vi "rename IPF.vi"(8 "error in":errorcluster, 9 "APG Config":T1, 10 "Programs List":i32(listbox), 11 "ref.Program List":refnum<vi>) -> (0 "error out":errorcluster, 2 "new filename":string)   [LabVIEW 2013, in "Manipulate IPF.lvlib"]
uses:
  Manipulate IPF.lvlib
  Settings/type_def/APG Config.ctl
  Pack Data/type_def/file types.ctl
  <userlib>/_OpenG.lib/file/file.llb/Strip Path Extension - 1D Array of Strings__ogtk.vi
  3013/code/Modules/GUI/GUI_5/subPanels/program/program.lvlib
  <userlib>/_OpenG.lib/file/file.llb/Convert File Extension (String)__ogtk.vi
  3013/code/a3Di.lvlib
  <userlib>/_OpenG.lib/file/file.llb/Convert File Extension (Path)__ogtk.vi
  Pack Data/Pack Files.lvlib
  Pack Data/type_def/command.ctl
  Settings/APG_settings.lvlib
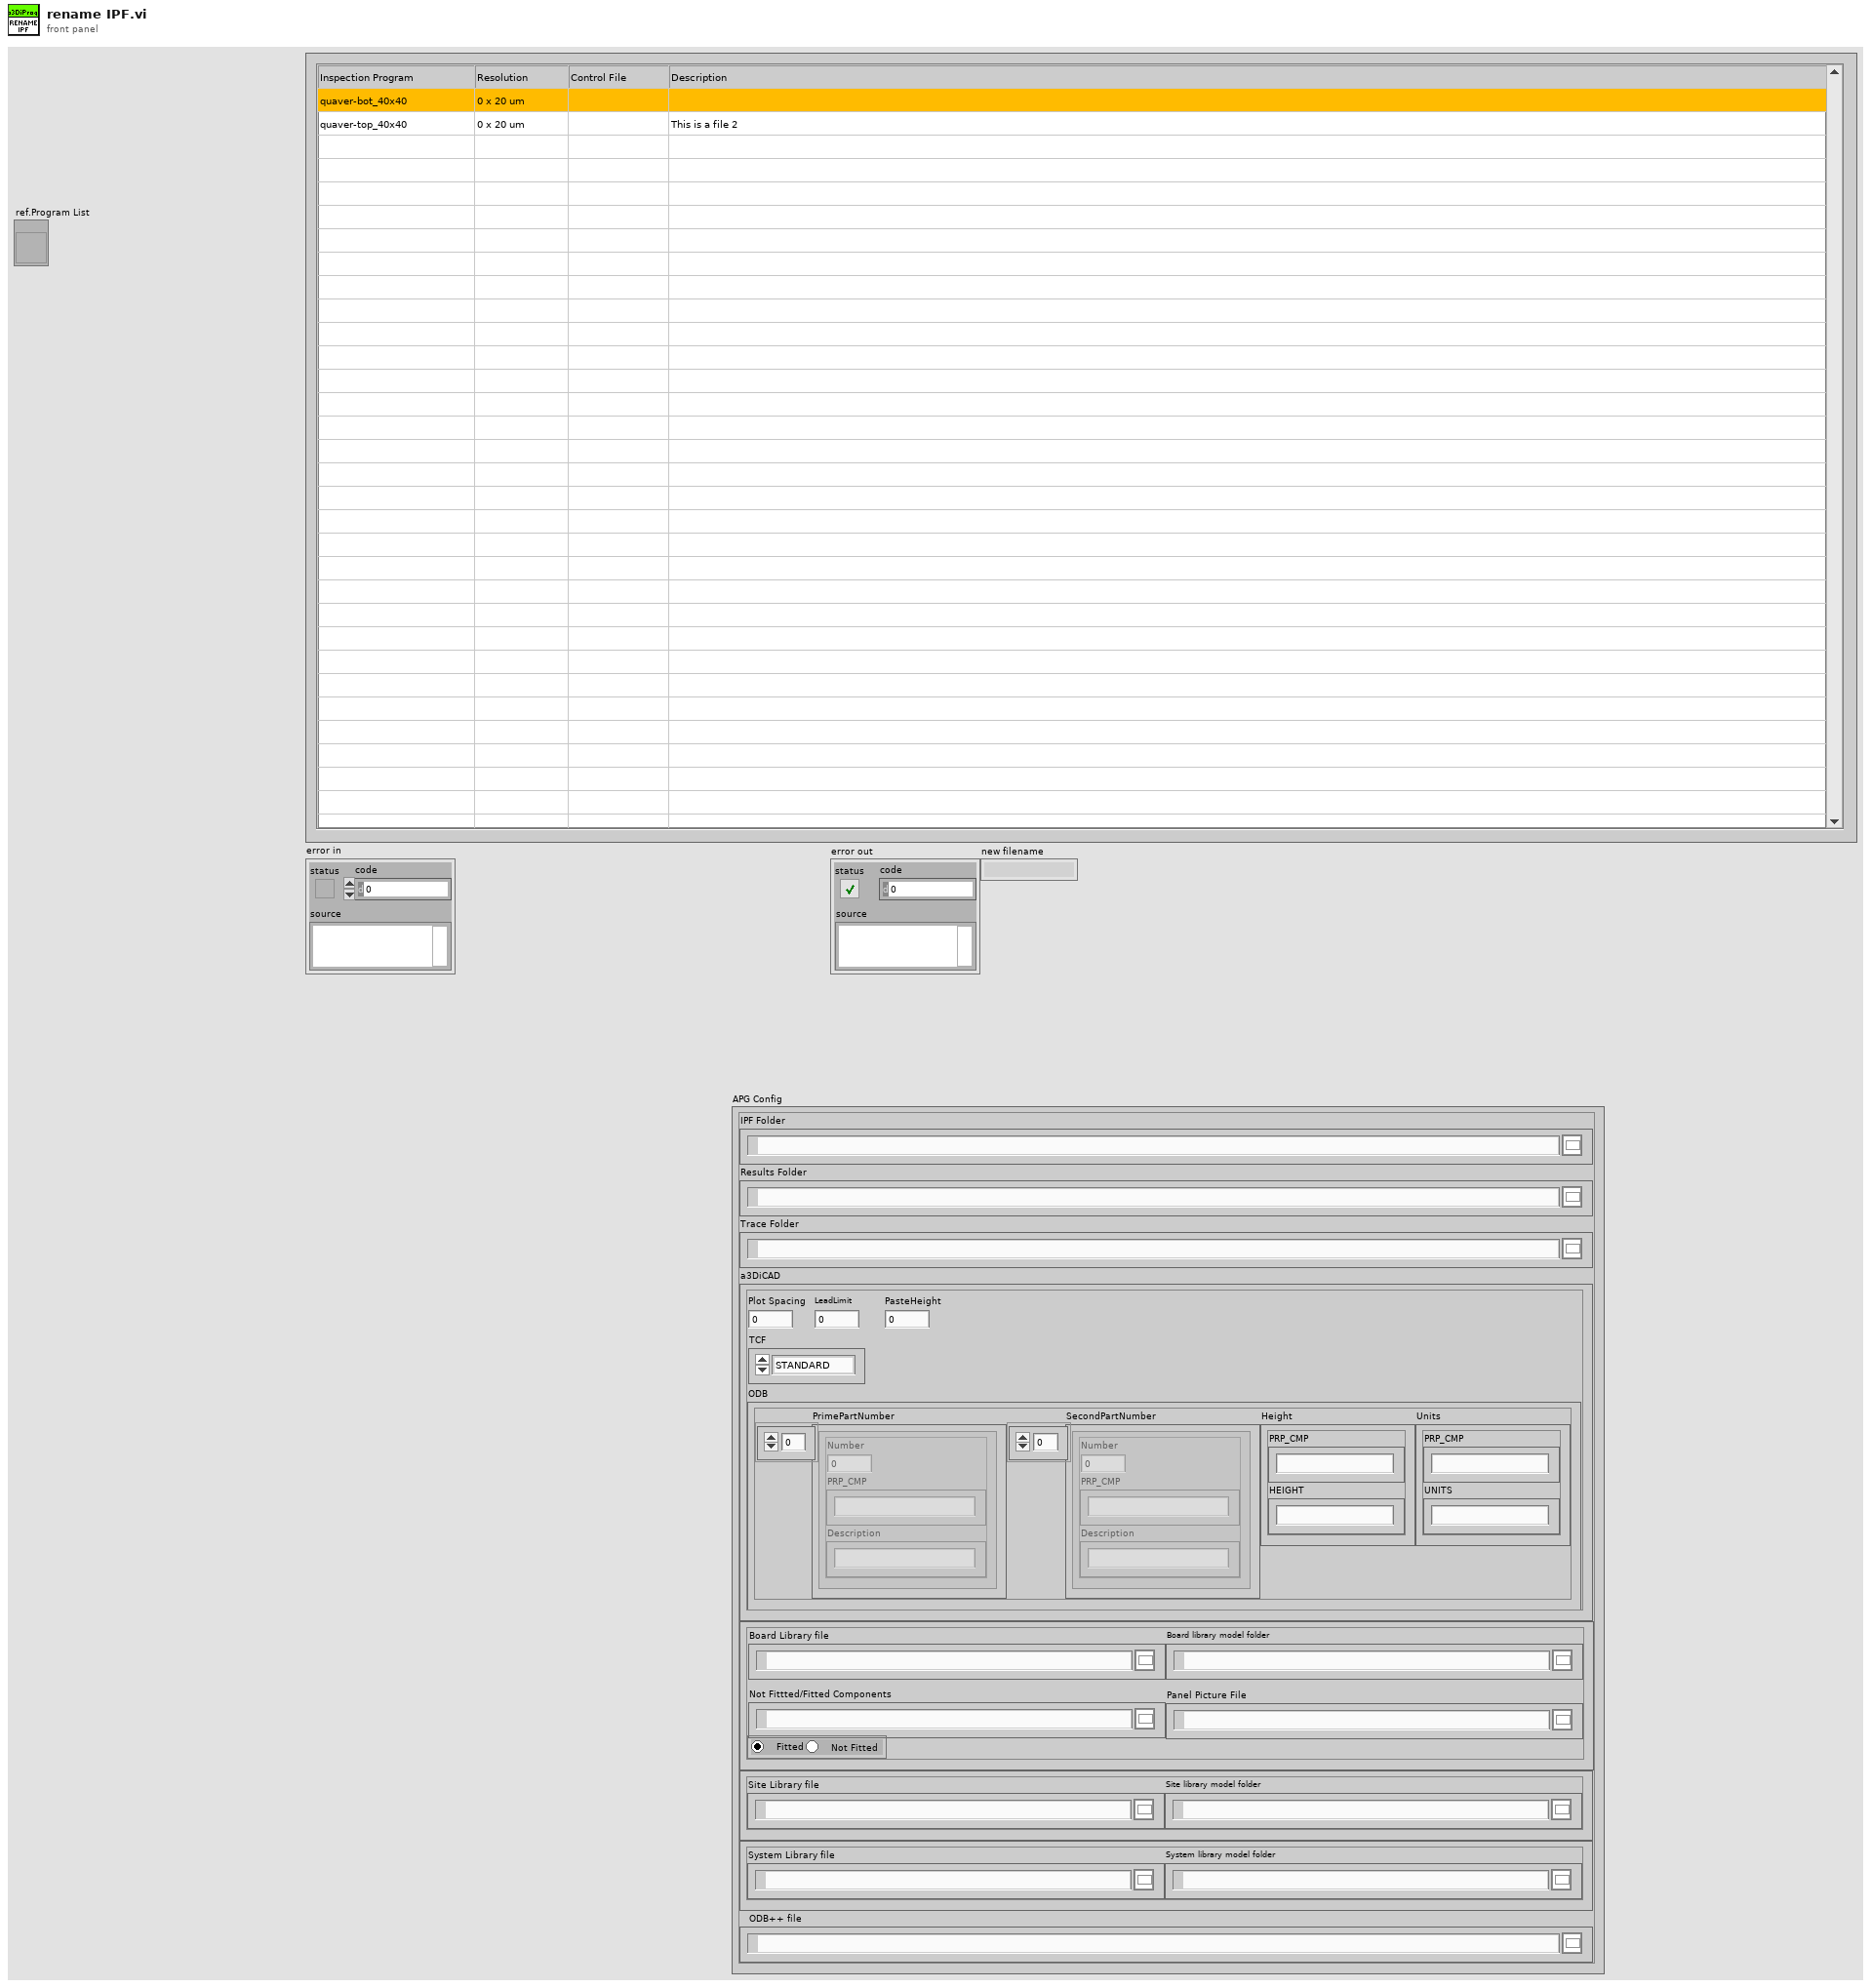
[diagram p1: front panel]
types:
  T1 = typedef "APG_settings.lvlib/APG Config.ctl" = cluster{"IPF Folder":path, "Results Folder":path, "Trace Folder":path, "a3DiCAD":cluster{"Plot Spacing":dbl, "TCF":enum16{"STANDARD", "PASTE", "LEAD"}, "LeadLimit":u32, "a3DiCADDebug":bool, "ODB":cluster{"PrimePartNumber":cluster{"Number":u32, "PRP_CMP":string, "Description":string}[], "SecondPartNumber":cluster{"Number":u32, "PRP_CMP":string, "Description":string}[], "Height":cluster{"PRP_CMP":string, "HEIGHT":string}, "Units":cluster{"PRP_CMP":string, "UNITS":string}}, "PasteHeight":dbl}, "a3DiCADcfg":path, "Board Library":cluster{"Board Library file":path, "Board library model folder":path, "Not Fittted/Fitted Components":path, "Panel Picture File":path, "Components":enum32{"Fitted", "Not Fitted "}}, "Site Library":cluster{"Site Library file":path, "Site library model folder":path}, "System Library":cluster{"System Library file":path, "System library model folder":path}, "ODB++ file":path}
  T2 = typedef "Pack Files.lvlib/file types.ctl" = enum16{"ODB", "TCF", "CAD Outline", "Config", "Inspection Prog", "a3Di-bin", "Results", "CAD Labels", "CAD Pads", "calScan_fid", "calScan_cal-tab", "PCB_SerialNumber", "CAD_Assembly", "Version", "Old Results", "CAD Picture", "Old TCF"}
  T3 = typedef "Pack Files.lvlib/command.ctl" = enum16{"Write", "Tar contents", "Read from Tar to File", "Delete", "Clean up Tar"}
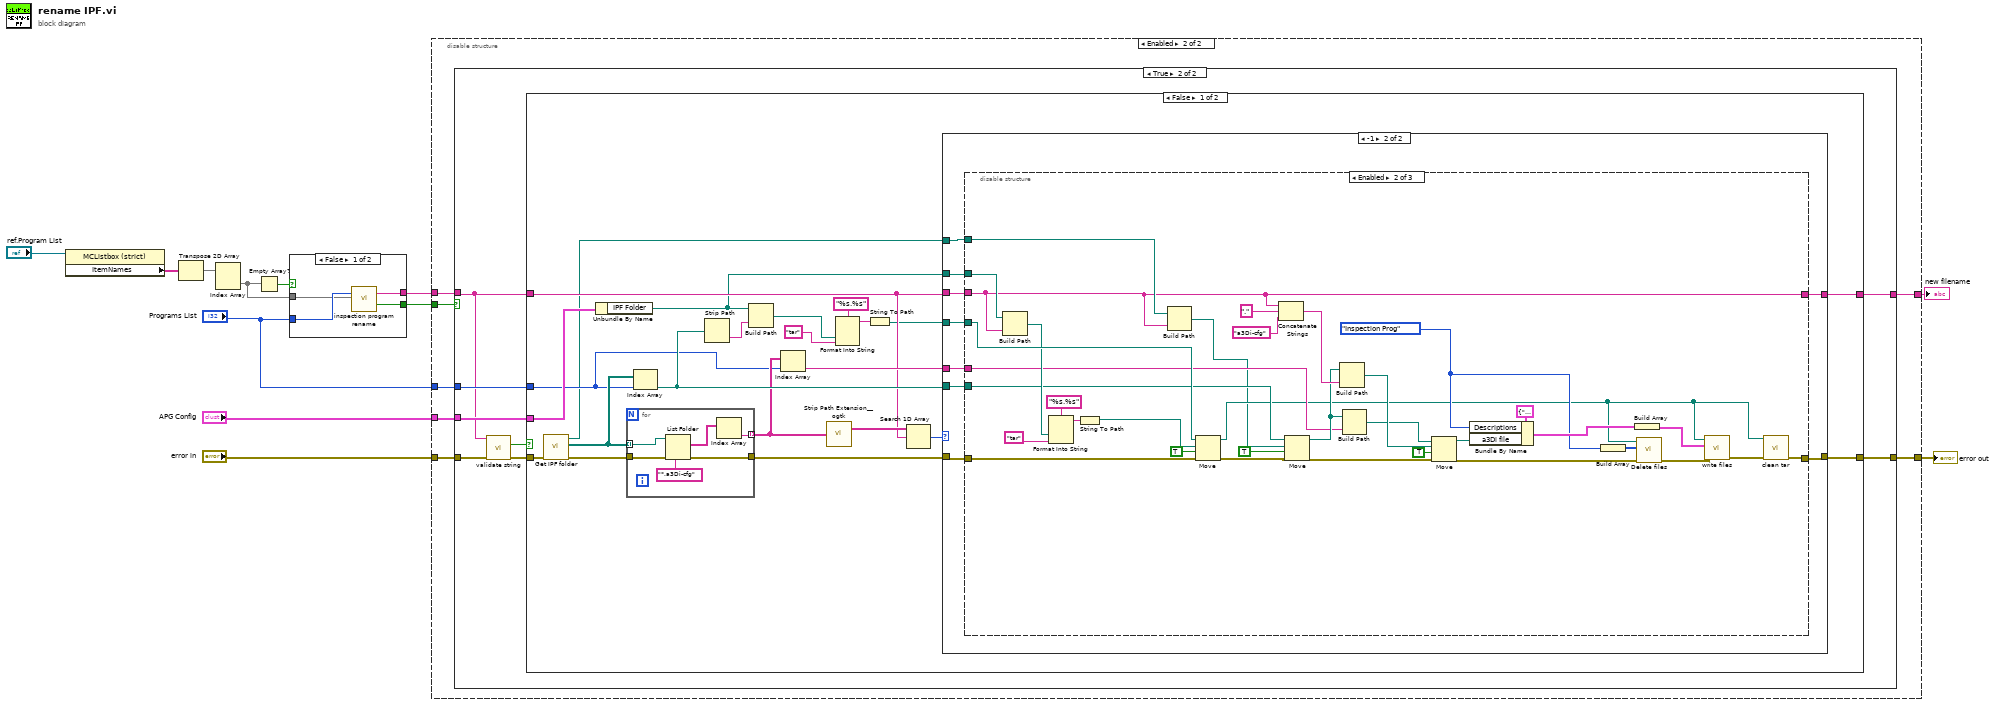
[diagram p0: block diagram]
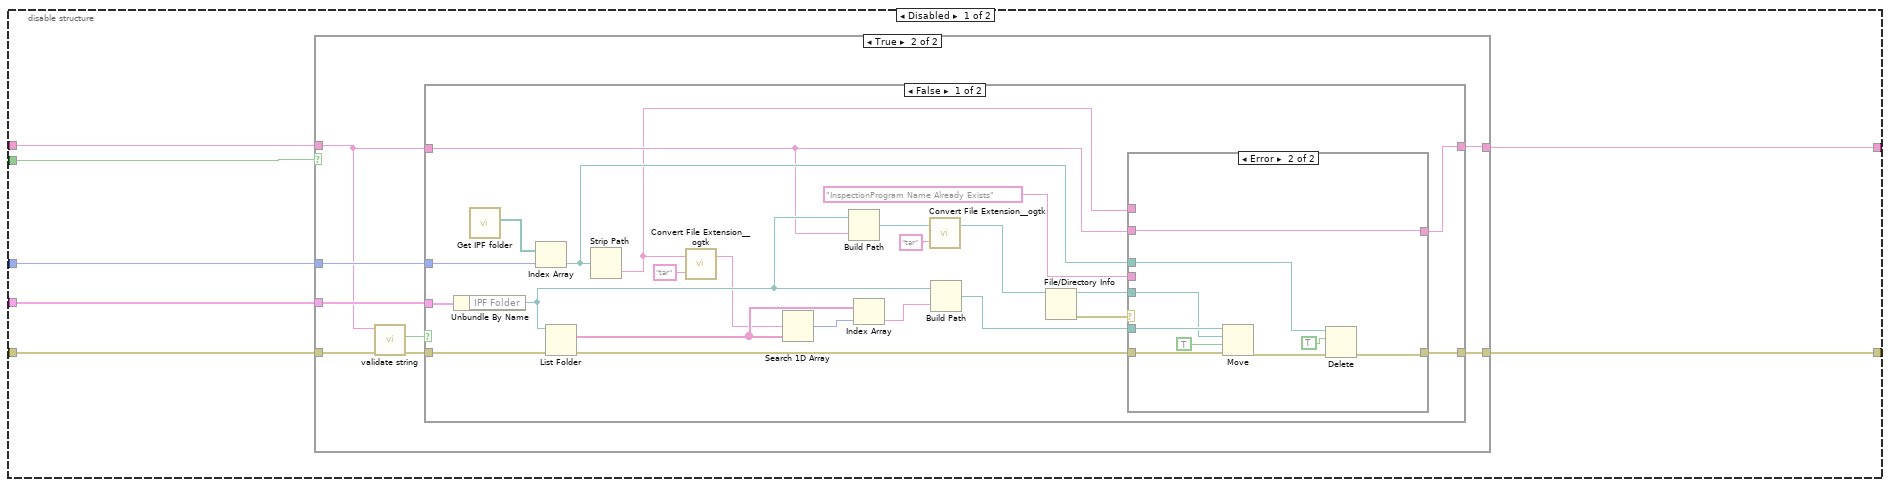
[diagram p2: hidden frame]
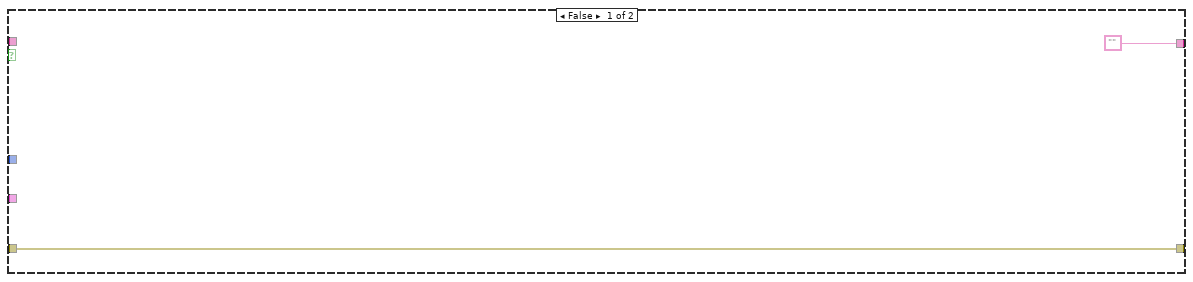
[diagram p3: hidden frame]
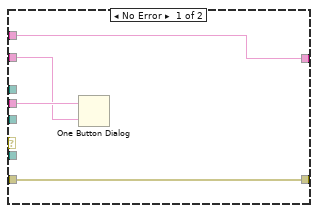
[diagram p4: hidden frame]
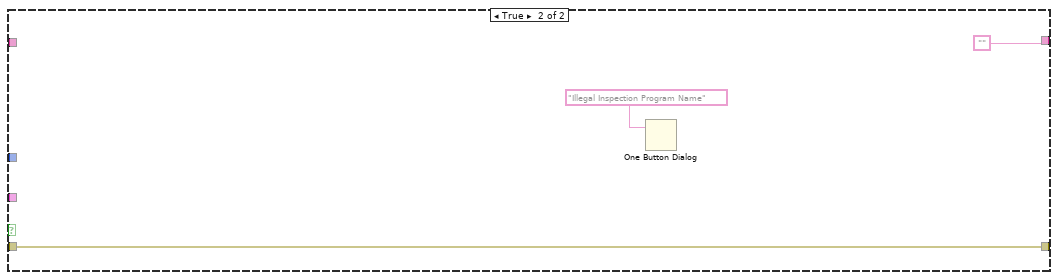
[diagram p5: hidden frame]
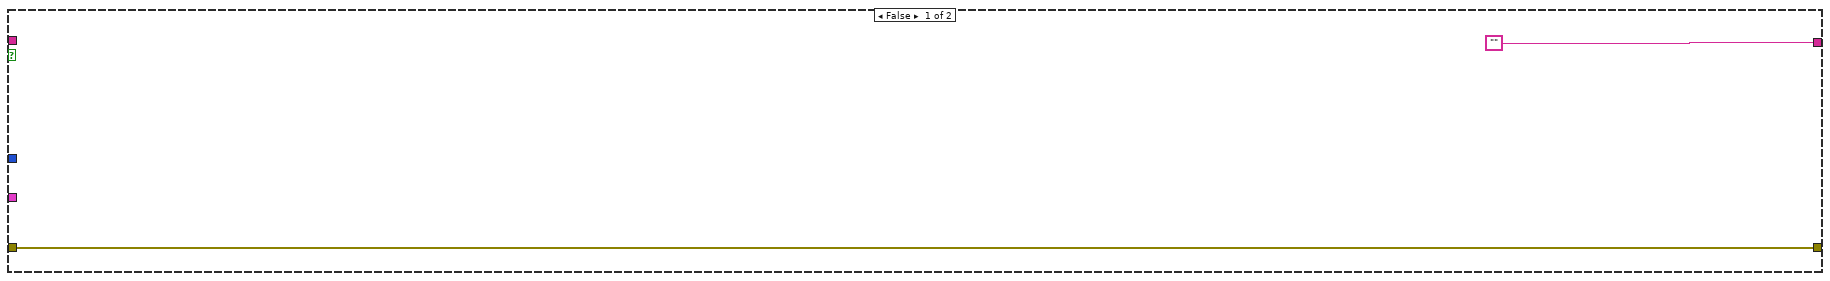
[diagram p6: hidden frame]
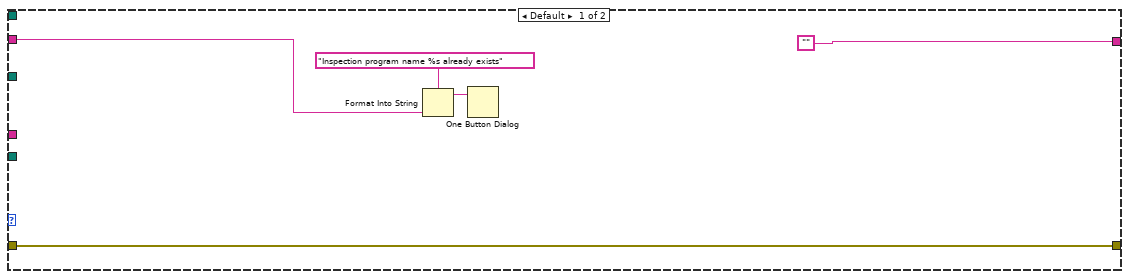
[diagram p7: hidden frame]
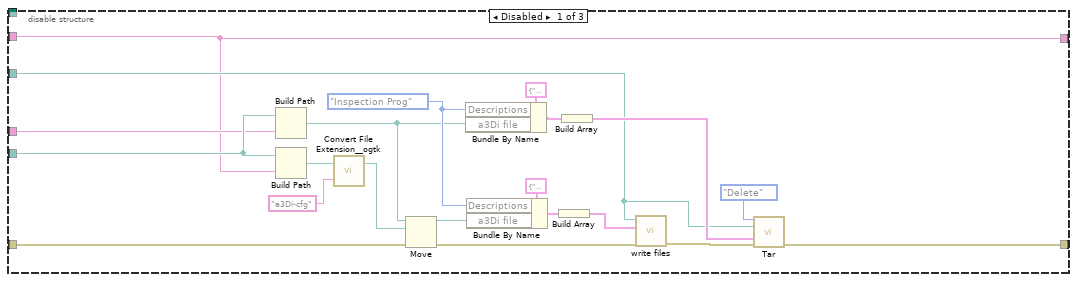
[diagram p8: hidden frame]
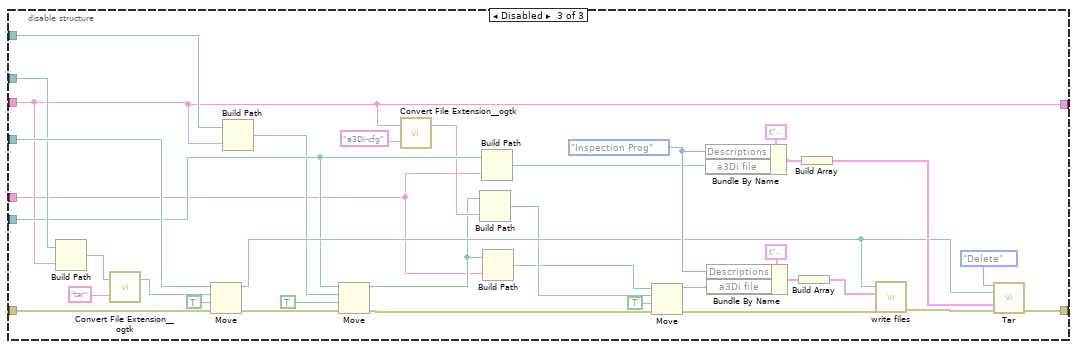
[diagram p9: hidden frame]
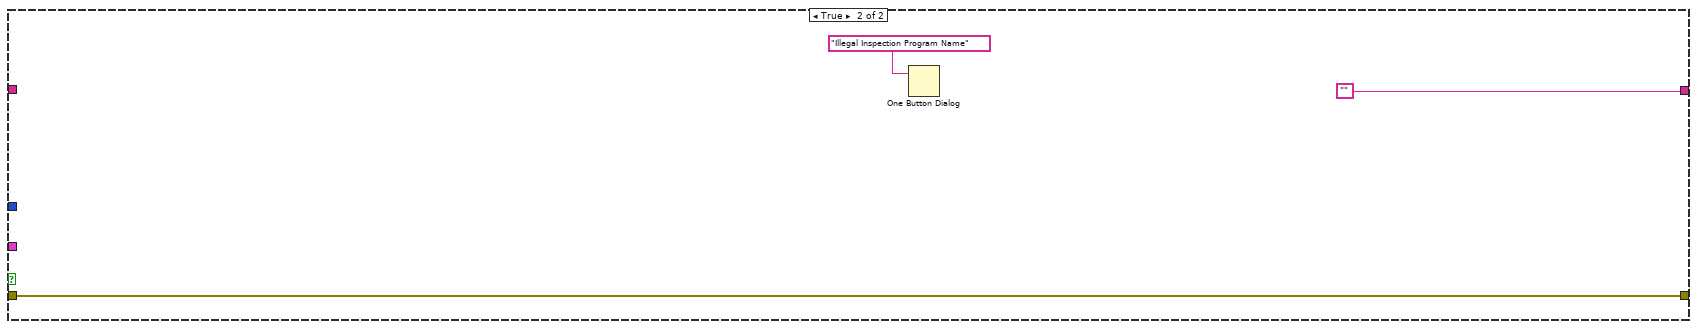
[diagram p10: hidden frame]
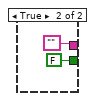
[diagram p11: hidden frame]
diagram:
  n1 = property class="MCListbox (strict)"(reference="ref.Program List") -> ("ItemNames"=w7:string[][])  [unwired: 1 in, 2 out]
  n2 = Transpose 2D Array(2D array=w7) -> (transposed array=w8:string[][])
  n3 = Index Array(array=w8) -> (element=w4:string[])  [unwired: 2 in]
  n4 = Empty Array?(array=w4) -> (empty?=w6:bool)
  n5 = case shown="False" w6 {
    tunnel: "Programs List" -> [w16 _]
    tunnel: w4 -> [w15 _]
    tunnel: [w14 FALSE ("OK")] -> w3
    tunnel: [w13 ""] -> w2
    frame False {
      n6 = call "inspection program rename.vi"("Selected Inspection Prog File Index"=w16, "Progs List[]"=w15) -> ("New Name"=w13:string, "OK"=w14:bool)  [unwired: 15 in, 1 out]
    }
    frame True {
    }
  }
  n7 = disable-structure shown="Enabled" {
    disable-tunnel: "error in" -> [w25 w81]
    disable-tunnel: [w24 w80] -> w11
    disable-tunnel: "APG Config" -> [w23 w79]
    disable-tunnel: "Programs List" -> [w22 w78]
    disable-tunnel: w3 -> [w21 w77]
    disable-tunnel: w2 -> [w20 w76]
    disable-tunnel: [w19 w75] -> w1
    frame Disabled {
      n8 = case shown="True" w21 {
        tunnel: w25 -> [w27 w33]
        tunnel: [w27 w35] -> w24
        tunnel: w23 -> [_ w32]
        tunnel: w22 -> [_ w34]
        tunnel: w20 -> [_ w29]
        tunnel: ["" w28] -> w19
        frame False {
        }
        frame True {
          n9 = call "validate string.vi"("error in (no error)"=w33, "String In"=w29) -> ("error out"=w30:errorcluster, "String Modified"=w31:bool)  [unwired: 6 in, 2 out]
          n10 = case shown="False" w31 {
            tunnel: [w58 w73] -> w35
            tunnel: w34 -> [w50 _]
            tunnel: w32 -> [w49 _]
            tunnel: w30 -> [w48 w73]
            tunnel: w29 -> [w38 _]
            tunnel: [w37 ""] -> w28
            frame False {
              n11 = Unbundle By Name(w49) -> ("IPF Folder"=w47:path)
              n12 = call "Get IPF folder.vi"() -> ("IPF sub folders"=w57:path[])  [unwired: 6 in, 5 out]
              n13 = Index Array(array=w57, index=w50) -> (element=w42:path)
              n14 = List Folder(path=w47, error in=w48) -> (filenames=w54:string[], error out=w55:errorcluster)  [unwired: 2 in, 2 out]
              n15 = Strip Path(path=w42) -> (name=w36:string)  [unwired: 1 out]
              n16 = call-poly <userlib>:"Convert File Extension__ogtk.vi"("new ending (none)"="tar", "file name"=w36) -> ("new filename"=w46:string)  [unwired: 1 out]
              n17 = Search 1D Array(1D array=w54, element=w46) -> (index of element=w56:i32)  [unwired: 1 in]
              n18 = Build Path(base path=w47, name or relative path=w38) -> (appended path=w40:path)
              n19 = Index Array(array=w54, index=w56) -> (element=w53:string)
              n20 = call-poly <userlib>:"Convert File Extension__ogtk.vi"("new ending (none)"="tar", "file name"=w40) -> ("new filename"=w39:path)  [unwired: 1 out]
              n21 = Build Path(base path=w47, name or relative path=w53) -> (appended path=w52:path)
              n22 = File/Directory Info(path=w39) -> (path out=w44:path, error out=w45:errorcluster)  [unwired: 1 in, 5 out]
              n23 = case shown="Error" w45 {
                tunnel: [w62 w66] -> w58
                tunnel: w55 -> [w62 w71]
                tunnel: w52 -> [_ w70]
                tunnel: w44 -> [_ w68]
                tunnel: "InspectionProgram Name Already Exists" ("message") -> [w61 _]
                tunnel: w42 -> [_ w64]
                tunnel: w38 -> [w59 w63]
                tunnel: [w60 w63] -> w37
                tunnel: w36 -> [w60 _]
                frame No Error {
                  n24 = One Button Dialog(message=w61, button name ("OK")=w59) -> ()  [unwired: 1 out]
                }
                frame Error {
                  n25 = Move(source path=w70, error in=w71, 9:TRUE ("overwrite (F)"), 10:w68) -> (error out=w67:errorcluster)  [unwired: 1 in, 2 out]
                  n26 = Delete(path (use dialog)=w64, entire hierarchy (F)=TRUE, error in=w67) -> (error out=w66:errorcluster)  [unwired: 2 in, 2 out]
                }
              }
            }
            frame True {
              n27 = One Button Dialog(message="Illegal Inspection Program Name") -> ()  [unwired: 1 in, 1 out]
            }
          }
        }
      }
    }
    frame Enabled {
      n28 = case shown="True" w77 {
        tunnel: w81 -> [w83 w89]
        tunnel: [w83 w91] -> w80
        tunnel: w79 -> [_ w88]
        tunnel: w78 -> [_ w90]
        tunnel: w76 -> [_ w85]
        tunnel: ["" w84] -> w75
        frame False {
        }
        frame True {
          n29 = call "validate string.vi"("error in (no error)"=w89, "String In"=w85) -> ("error out"=w86:errorcluster, "String Modified"=w87:bool)  [unwired: 6 in, 2 out]
          n30 = case shown="False" w87 {
            tunnel: [w105 w226] -> w91
            tunnel: w90 -> [w101 _]
            tunnel: w88 -> [w113 _]
            tunnel: w86 -> [w108 w226]
            tunnel: w85 -> [w99 _]
            tunnel: [w112 ""] -> w84
            frame False {
              n31 = call "Get IPF folder.vi"("error in (no error)"=w108) -> ("error out"=w107:errorcluster, "IPF sub folders"=w111:path[], "IPF Folder"=w97:path)  [unwired: 5 in, 3 out]
              n32 = Unbundle By Name(w113) -> ("IPF Folder"=w98:path)
              n33 = for {
                tunnel: w111 -> [w117] mode=indexing
                tunnel: [w116] -> w102 mode=indexing
                tunnel: w107 -> [w115]
                tunnel: [w114] -> w106
                n34 = List Folder(path=w117, pattern="*.a3Di-cfg", error in=w115) -> (filenames=w118:string[], error out=w114:errorcluster)  [unwired: 1 in, 2 out]
                n35 = Index Array(array=w118) -> (element=w116:string)  [unwired: 1 in]
              }
              n36 = Index Array(array=w111, index=w101) -> (element=w104:path)
              n37 = Strip Path(path=w104) -> (name=w103:string)  [unwired: 1 out]
              n38 = Build Path(base path=w98, name or relative path=w103) -> (appended path=w94:path)
              n39 = Index Array(array=w102, index=w101) -> (element=w100:string)
              n40 = call-poly <userlib>:"Strip Path Extension__ogtk.vi"("paths"=w102) -> ("roots"=w109:string[])  [unwired: 1 out]
              n41 = Format Into String(format string="%s.%s", w94, "tar" ("new ending (none)")) -> (resulting string=w93:string)  [unwired: 2 in, 1 out]
              n42 = String To Path(string=w93) -> (path=w95:path)
              n43 = Search 1D Array(1D array=w109, element=w99) -> (index of element=w110:i32)  [unwired: 1 in]
              n44 = case shown="-1" w110 {
                tunnel: w104 -> [_ w132]
                tunnel: w99 -> [w122 w128]
                tunnel: ["" w127] -> w112
                tunnel: w106 -> [w124 w133]
                tunnel: [w124 w131] -> w105
                tunnel: w95 -> [_ w130]
                tunnel: w100 -> [_ w129]
                tunnel: w98 -> [_ w126]
                tunnel: w97 -> [_ w125]
                frame Default {
                  n45 = Format Into String(format string="Inspection program name %s already exists" ("message"), w122) -> (resulting string=w121:string)  [unwired: 2 in, 1 out]
                  n46 = One Button Dialog(message=w121) -> ()  [unwired: 1 in, 1 out]
                }
                frame -1 {
                  n47 = disable-structure shown="Enabled" {
                    disable-tunnel: w133 -> [w154 w185 w213]
                    disable-tunnel: w132 -> [w153 w176 w203]
                    disable-tunnel: [w150 w161 w223] -> w131
                    disable-tunnel: w130 -> [w143 w182 w210]
                    disable-tunnel: w129 -> [w138 w167 w190]
                    disable-tunnel: w128 -> [w134 w171 w194]
                    disable-tunnel: [w134 w171 w194] -> w127
                    disable-tunnel: w126 -> [_ w181 w209]
                    disable-tunnel: w125 -> [_ w180 w208]
                    frame Disabled {
                      w141 = file_types."Inspection Prog" ("Descriptions")
                      n48 = Build Path(base path=w153, name or relative path=w138) -> (appended path=w139:path)
                      n49 = Build Path(base path=w153, name or relative path=w134) -> (appended path=w136:path)
                      n50 = call-poly <userlib>:"Convert File Extension__ogtk.vi"("new ending (none)"="a3Di-cfg", "file name"=w136) -> ("new filename"=w135:path)  [unwired: 1 out]
                      n51 = Move(source path=w139, error in=w154, 10:w135) -> (error out=w152:errorcluster, 3:w142:path)  [unwired: 2 in, 1 out]
                      n52 = Bundle By Name(cluster=cluster{"Descriptions":T2, "a3Di file":path} {"Descriptions"=enum."ODB", "a3Di file"=path ""} ("Cluster"), "Descriptions"=w141, "a3Di file"=w139) -> (w140:cluster{"Descriptions":T2, "a3Di file":path})
                      n53 = Bundle By Name(cluster=cluster{"Descriptions":T2, "a3Di file":path} {"Descriptions"=enum."ODB", "a3Di file"=path ""} ("Cluster"), "Descriptions"=w141, "a3Di file"=w142) -> (w146:cluster{"Descriptions":T2, "a3Di file":path})
                      n54 = Build Array(w146) -> (w144:cluster{"Descriptions":T2, "a3Di file":path}[])
                      n55 = Build Array(w140) -> (w145:cluster{"Descriptions":T2, "a3Di file":path}[])
                      n56 = call "write files.vi"("error in (no error)"=w152, "Files to be zipped"=w144, "a3Di  tar file"=w143) -> ("error out"=w151:errorcluster)  [unwired: 7 in, 1 out]
                      n57 = call "Tar.vi"("Command"=command."Delete", "a3Di  tar file"=w143, "a3Di Files"=w145, "error in (no error)"=w151) -> ("error out"=w150:errorcluster)  [unwired: 8 in, 3 out]
                    }
                    frame Enabled {
                      w164 = file_types."Inspection Prog" ("Descriptions")
                      n58 = Build Path(base path=w181, name or relative path=w171) -> (appended path=w179:path)
                      n59 = Format Into String(format string="%s.%s", w179, "tar" ("new ending (none)")) -> (resulting string=w156:string)  [unwired: 2 in, 1 out]
                      n60 = String To Path(string=w156) -> (path=w178:path)
                      n61 = Build Path(base path=w180, name or relative path=w171) -> (appended path=w159:path)
                      n62 = Move(source path=w182, error in=w185, 9:TRUE ("overwrite (F)"), 10:w178) -> (error out=w186:errorcluster, 3:w160:path)  [unwired: 1 in, 1 out]
                      n63 = Concatenate Strings(w171, "." ("string"), "a3Di-cfg" ("new ending (none)")) -> (w170:string)
                      n64 = Move(source path=w176, error in=w186, 9:TRUE ("overwrite (F)"), 10:w159) -> (error out=w175:errorcluster, 3:w168:path)  [unwired: 1 in, 1 out]
                      n65 = Build Path(base path=w168, name or relative path=w170) -> (appended path=w173:path)
                      n66 = Build Path(base path=w168, name or relative path=w167) -> (appended path=w169:path)
                      n67 = Move(source path=w169, error in=w175, 9:TRUE ("overwrite (F)"), 10:w173) -> (error out=w166:errorcluster, 3:w174:path)  [unwired: 1 in, 1 out]
                      n68 = Bundle By Name(cluster=cluster{"Descriptions":T2, "a3Di file":path} {"Descriptions"=enum."ODB", "a3Di file"=path ""} ("Cluster"), "Descriptions"=w164, "a3Di file"=w174) -> (w188:cluster{"Descriptions":T2, "a3Di file":path})
                      n69 = Build Array(w164) -> (w163:T2[])
                      n70 = Build Array(w188) -> (w187:cluster{"Descriptions":T2, "a3Di file":path}[])
                      n71 = call "Delete files.vi"("error in (no error)"=w166, "File type[]"=w163, "a3Di  tar file"=w160) -> ("error out"=w165:errorcluster)  [unwired: 8 in]
                      n72 = call "write files.vi"("error in (no error)"=w165, "Files to be zipped"=w187, "a3Di  tar file"=w160) -> ("error out"=w162:errorcluster)  [unwired: 7 in, 1 out]
                      n73 = call "clean tar.vi"("tar file"=w160, "error in (no error)"=w162) -> ("error out"=w161:errorcluster)  [unwired: 13 in]
                    }
                    frame Disabled {
                      w216 = file_types."Inspection Prog" ("Descriptions")
                      n74 = Build Path(base path=w209, name or relative path=w194) -> (appended path=w206:path)
                      n75 = call-poly <userlib>:"Convert File Extension__ogtk.vi"("new ending (none)"="tar", "file name"=w206) -> ("new filename"=w205:path)  [unwired: 1 out]
                      n76 = Move(source path=w210, error in=w213, 9:TRUE ("overwrite (F)"), 10:w205) -> (error out=w214:errorcluster, 3:w207:path)  [unwired: 1 in, 1 out]
                      n77 = Build Path(base path=w208, name or relative path=w194) -> (appended path=w202:path)
                      n78 = Move(source path=w203, error in=w214, 9:TRUE ("overwrite (F)"), 10:w202) -> (error out=w201:errorcluster, 3:w191:path)  [unwired: 1 in, 1 out]
                      n79 = call-poly <userlib>:"Convert File Extension__ogtk.vi"("new ending (none)"="a3Di-cfg", "file name"=w194) -> ("new filename"=w193:string)  [unwired: 1 out]
                      n80 = Build Path(base path=w191, name or relative path=w193) -> (appended path=w198:path)
                      n81 = Build Path(base path=w203, name or relative path=w190) -> (appended path=w196:path)
                      n82 = Build Path(base path=w191, name or relative path=w190) -> (appended path=w192:path)
                      n83 = Move(source path=w192, error in=w201, 9:TRUE ("overwrite (F)"), 10:w198) -> (error out=w200:errorcluster, 3:w199:path)  [unwired: 1 in, 1 out]
                      n84 = Bundle By Name(cluster=cluster{"Descriptions":T2, "a3Di file":path} {"Descriptions"=enum."ODB", "a3Di file"=path ""} ("Cluster"), "Descriptions"=w216, "a3Di file"=w196) -> (w215:cluster{"Descriptions":T2, "a3Di file":path})
                      n85 = Bundle By Name(cluster=cluster{"Descriptions":T2, "a3Di file":path} {"Descriptions"=enum."ODB", "a3Di file"=path ""} ("Cluster"), "Descriptions"=w216, "a3Di file"=w199) -> (w219:cluster{"Descriptions":T2, "a3Di file":path})
                      n86 = Build Array(w219) -> (w217:cluster{"Descriptions":T2, "a3Di file":path}[])
                      n87 = Build Array(w215) -> (w218:cluster{"Descriptions":T2, "a3Di file":path}[])
                      n88 = call "write files.vi"("error in (no error)"=w200, "Files to be zipped"=w217, "a3Di  tar file"=w207) -> ("error out"=w224:errorcluster)  [unwired: 7 in, 1 out]
                      n89 = call "Tar.vi"("Command"=command."Delete", "a3Di  tar file"=w207, "a3Di Files"=w218, "error in (no error)"=w224) -> ("error out"=w223:errorcluster)  [unwired: 8 in, 3 out]
                    }
                  }
                }
              }
            }
            frame True {
              n90 = One Button Dialog(message="Illegal Inspection Program Name") -> ()  [unwired: 1 in, 1 out]
            }
          }
        }
      }
    }
  }
  "error out" <- w11
  "new filename" <- w1
